vi "Do.vi"(8 "error in (no error)":errorcluster, 10 "Boxes":map{i32, string[]}(c390), 11 "Proto in":refnum<class "Proto.lvclass">) -> (0 "error out":errorcluster, 2 "Boxes out":map{i32, string[]}(c390), 3 "Proto out":refnum<class "Proto.lvclass">)   [LabVIEW 2021, in "Proto.lvclass"]
uses:
  Proto.lvclass
  Proto.lvclass/Proto.ctl
  <vilib>/Utility/miscctls.llb/LVMapReplaceAction.ctl
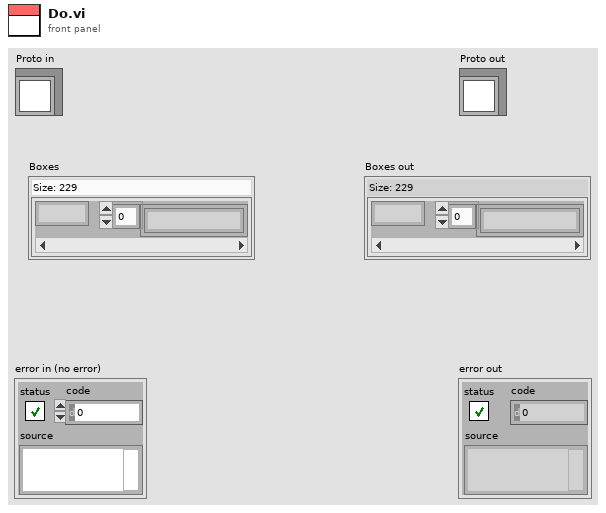
[diagram p1: front panel]
types:
  T1 = typedef "LVMapReplaceAction.ctl" = enum32{"Modify Entry only if found", "Add or Modify Entry", "Delete Entry"}
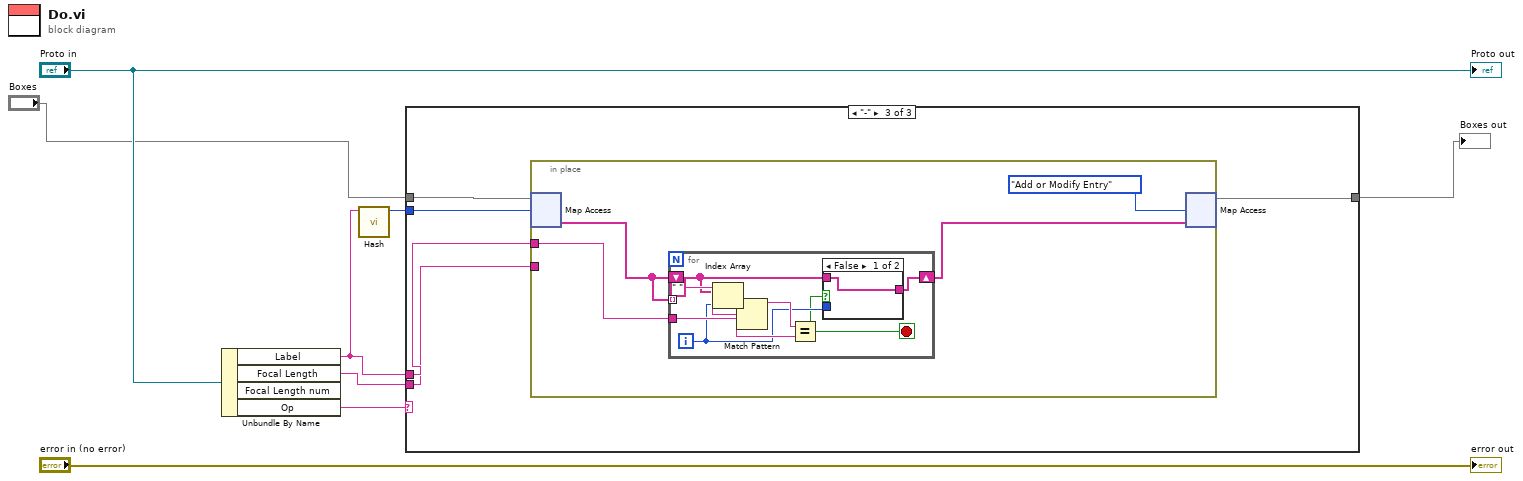
[diagram p0: block diagram]
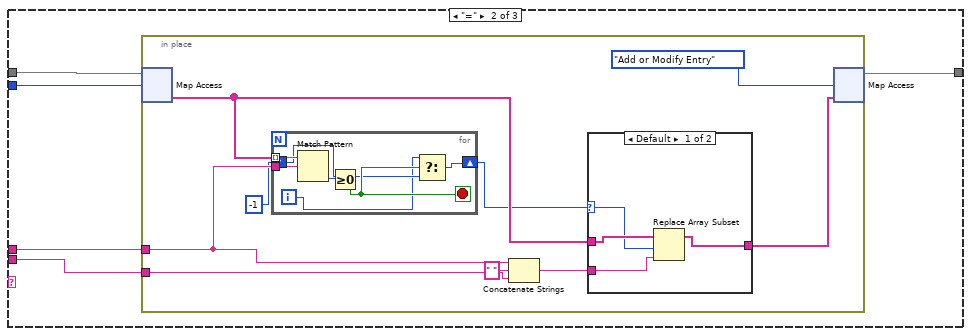
[diagram p3: hidden frame]
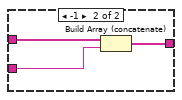
[diagram p4: hidden frame]
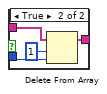
[diagram p5: hidden frame]
diagram:
  n1 = Unbundle By Name("Proto in") -> ("Label"=w2:string, "Focal Length"=w3:string, "Op"=w4:string)  [unwired: 1 out]
  n2 = call "Hash.vi"("String"=w2) -> ("Numeric"=w1:u64)  [unwired: 10 in]
  n3 = case shown="\"-\"" w4 {
    tunnel: "Boxes" -> [w9 w14 w42]
    tunnel: [w9 w13 w41] -> w5
    tunnel: w1 -> [_ w12 w40]
    tunnel: w2 -> [_ w11 w39]
    tunnel: w3 -> [_ w10 w38]
    frame Default {
    }
    frame "=" {
      n4 = in-place {
        in-place-border: w11 -> [w17]
        in-place-border: w10 -> [w19]
        n5 = in-place-map #1(w14, w12) -> (w18:string[])  [unwired: 1 in, 1 out]
        n6 = for {
          tunnel: w18 -> [w37] mode=indexing
          tunnel: w17 -> [w36]
          shift-right: [w34] -> w15
          shift-left: -1 -> [w32]
          i -> [w31]
          stop <- w33 stop-if-true
          n7 = Match Pattern(string=w37, regular expression=w36) -> (offset past match=w35:i32)  [unwired: 1 in, 3 out]
          n8 = Greater Or Equal To 0?(x=w35) -> (x >= 0?=w33:bool)
          n9 = Select(t=w31, s=w33, f=w32) -> (s? t:f=w34:i32)
        }
        n10 = Concatenate Strings(w17, " " ("string"), w19) -> (w21:string)
        n11 = case shown="Default" w15 {
          selector: w15 -> [w26 _]
          tunnel: [w24 w30] -> w22
          tunnel: w21 -> [w25 w29]
          tunnel: w18 -> [w27 w28]
          frame Default {
            n12 = Replace Array Subset(array=w27, new element=w25, index=w26) -> (w24:string[])
          }
          frame -1 {
            n13 = Build Array (concatenate)(w28, w29) -> (w30:string[])
          }
        }
        n14 = in-place-map #1(w22, LVMapReplaceAction."Add or Modify Entry" ("action")) -> (w13:map{i32, string[]})  [unwired: 2 out]
      }
    }
    frame "-" {
      n15 = in-place {
        in-place-border: w39 -> [w45]
        in-place-border: w38 -> [_]
        n16 = in-place-map #2(w42, w40) -> (w43:string[])  [unwired: 1 in, 1 out]
        n17 = for {
          tunnel: w45 -> [w52]
          shift-right: [w49] -> w44
          shift-left: w43 -> [w50]
          tunnel: w43 -> [_] mode=indexing
          i -> [w48]
          stop <- w47 stop-if-true
          n18 = Index Array(array=w50, index=w48) -> (element=w51:string)
          n19 = Match Pattern(string=w51, regular expression=" ") -> (before substring=w54:string)  [unwired: 1 in, 3 out]
          n20 = Equal?(x=w54, y=w52) -> (x = y?=w47:bool)
          n21 = case shown="False" w47 {
            tunnel: w50 -> [w55 w59]
            tunnel: [w55 w58] -> w49
            tunnel: w48 -> [_ w57]
            frame False {
            }
            frame True {
              n22 = Delete From Array(array=w59, length=1, index=w57) -> (array with subset deleted=w58:string[])  [unwired: 1 out]
            }
          }
        }
        n23 = in-place-map #2(w44, LVMapReplaceAction."Add or Modify Entry" ("action")) -> (w41:map{i32, string[]})  [unwired: 2 out]
      }
    }
  }
  "Boxes out" <- w5
  "error out" <- "error in (no error)"
  "Proto out" <- "Proto in"
